vi "Main.vi"() -> ()   [LabVIEW 2018]
uses:
  <vilib>/addons/database/Connection.llb/DB Tools Open Connec (String).vi
  <vilib>/addons/database/NI_Database_API.lvlib
  <vilib>/ptbypt/NI_PtbyPt.lvlib
panel:
  out "元素":cluster{"Data":string[], "State":T1}
  out "Code":string
  out "退出":bool
  out "Main Tab":T2(tab)
  out "ST80通讯状态":bool caption="ST60通讯状态"
  in  "错误信息":i32(listbox)
  out "ST30通讯状态":bool caption="ST10通讯状态"
  out "ST50通讯状态":bool
  out "ST70通讯状态":bool caption="ST60通讯状态"
  out "ST60通讯状态":bool caption="ST70通讯状态"
  out "ST40通讯状态":bool
  out "ST20通讯状态":bool
  out "ST10通讯状态":bool
  in  "每工站主要显示":T3(tab)
  in  "ST10-2_DATA":i32(listbox) caption="ST10_DATA"
  in  "ST10-1_DATA":i32(listbox) caption="ST10_DATA"
  in  "ST20-3_DATA":i32(listbox) caption="ST20_DATA"
  in  "ST20-2_DATA":i32(listbox) caption="ST20_DATA"
  in  "ST30-2_DATA":i32(listbox) caption="ST20_DATA"
  in  "ST30-1_DATA":i32(listbox) caption="ST20_DATA"
  in  "ST40-3_DATA":i32(listbox) caption="ST20_DATA"
  in  "ST40-1_DATA":i32(listbox) caption="ST20_DATA"
  in  "ST50-3_DATA":i32(listbox) caption="ST20_DATA"
  in  "ST50-2_DATA":i32(listbox) caption="ST20_DATA"
  in  "ST60-2_DATA":i32(listbox) caption="ST20_DATA"
  in  "ST60-1_DATA":i32(listbox) caption="ST20_DATA"
  in  "ST70_DATA":i32(listbox) caption="ST20_DATA"
  out "XY图":cluster{"X":dbl, "Y":dbl}[](graph)
  in  "登录界面":bool
  in  "注销":bool
  in  "修改密码":bool
  in  "Rework界面":bool
  out "产品型号":string
  in  "界面切换":bool
  in  "登录界面返回":bool
  out "登录状态":string
  in  "登录":bool
  in  "输入管理员密码":string
  in  "修改密码界面返回":bool
  out "修改密码状态":string
  in  "确认修改密码":bool
  in  "新密码":string
  in  "初始密码":string
  in  "80":bool
  in  "602":bool
  in  "403":bool
  in  "302":bool
  in  "203":bool
  in  "101":bool
  out "Rework状态":string
  in  "查询":bool
  in  "确定Rework":bool
  in  "Rework返回":bool
  in  "输入需要Rework的一维码：":string
  in  "102":bool
  in  "202":bool
  in  "301":bool
  in  "401":bool
  in  "502":bool
  in  "503":bool
  in  "601":bool
  in  "70":bool
  in  "Monitor Tab":T4(tab)
  out "202读取数据":string[](array[string])
  out "ST102数据读取（事件）":bool
  out "ST10 Shaft M0102049":string caption="ST101 Shaft M0102049"
  out "数据保存请求回复101":string
  out "扫码请求回复102":string
  out "上一站结果(102)":string
  out "上一站号(102)":string
  out "ST102扫码请求":bool
  out "ST101扫码请求":bool
  out "ST101数据读取":bool
  out "扫码请求回复101":string
  in  "ST102扫码请求（事件）":bool
  out "ST101扫码请求（事件）":bool
  out "ST101数据读取（事件）":bool
  in  "返回":bool
  out "ST102数据读取":bool
  out "数据保存请求回复102":string
  out "101 二维码":string
  out "102 二维码":string
  out "ST10 Form Seal 5026859":string caption="ST101 Form Seal 5026859"
  out "ST10 Dowel Pin 5024532":string caption="ST101 Dowel Pin 5024532"
  out "ST10 Flange M0104918":string caption="ST101 Flange M0104918"
  out "ST10 Control Plat 5025303":string caption="ST101 Control Plat 5025303"
  out "ST10 Dowel Pin 5020281":string caption="ST101 Dowel Pin 5020281"
  out "ST203扫码请求":bool
  out "202二维码":string caption="203二维码"
  out "ST203扫码请求（事件）":bool
  out "扫码请求回复202":string caption="扫码请求回复203"
  out "ST202数据读取":bool caption="ST203数据读取"
  out "ST203数据读取（事件）":bool
  out "数据保存请求回复202":string caption="数据保存请求回复203"
  out "ST202 Dowel Pin M0104893":string caption="ST20 Dowel Pin M0104893"
  out "ST202 Camring 5026187":string caption="ST20 Camring 5026187"
  out "ST202 Rotor 5025805":string caption="ST20 Rotor 5025805"
  out "201二维码":string caption="202二维码"
  out "上一站号 (202)":string
  out "上一站结果 (202)":string
  out "扫码请求回复201":string caption="扫码请求回复202"
  out "数据保存请求回复201":string caption="数据保存请求回复202"
  out "ST201数据读取":bool caption="ST202数据读取"
  out "ST202扫码请求":bool
  out "ST202扫码请求(事件)":bool
  in  "ST202数据读取(事件)":bool
  out "上一站结果 (203)":string
  out "上一站号 (203)":string
  out "State 10":T1
  out "10":i32
  out "20":i32
  out "20 State":T1
  out "101 上一站号":string
  out "101 上一站结果":string
  out "102读取数据":string[](array[string])
  out "数据库连接状态":string="连接成功"
  out "403读取数据":string[](array[string])
  out "302读取数据":string[](array[string])
  out "301 二维码":string
  out "302 二维码":string
  out "ST301扫码请求":bool
  out "上一站号 (301)":string
  out "上一站结果 (301)":string
  out "ST301数据读取 (事件)":bool
  out "ST301扫码请求 (事件)":bool
  out "ST302数据读取 (事件)":bool
  out "ST302扫码请求 (事件)":bool
  out "扫码请求回复301":string
  out "ST301数据读取":bool
  out "数据保存请求回复301":string
  out "ST302扫码请求":bool
  out "扫码请求回复302":string
  out "ST302数据读取":bool
  out "ST301 Vane 5004737":string caption="ST30 Vane 5004737"
  out "ST301 Dowel Pin 5024533":string caption="ST30 Dowel Pin 5024533"
  out "ST301 Dowel Pin 5020282":string caption="ST30 Dowel Pin 5020282"
  out "数据保存请求回复302":string
  out "401二维码":string
  out "402二维码 2":string caption="402二维码"
  out "403二维码":string
  out "ST401扫码请求":bool
  out "扫码请求回复401":string
  out "ST401数据读取":bool
  out "数据保存请求回复401":string
  out "ST402扫码请求":bool
  out "扫码请求回复402":string
  out "ST402数据读取":bool
  out "数据保存请求回复402":string
  out "ST403扫码请求":bool
  out "扫码请求回复403":string
  out "ST403数据读取":bool
  out "数据保存请求回复403":string
  out "ST403数据读取（事件）":bool
  out "ST403扫码请求(事件)":bool
  out "ST401数据读取（事件）":bool
  out "ST401扫码请求(事件)":bool
  out "ST402数据读取（事件）":bool
  out "ST402扫码请求(事件)":bool caption="ST402扫码请求（事件）"
  out "上一站号 (401)":string
  out "上一站结果 (401)":string
  out "ST40 Circlip 5026621":string
  out "上一站结果 (302)":string
  out "上一站号 (302)":string
  out "上一站结果 (403)":string
  out "上一站号 (403)":string
  out "30_State":T1
  out "30":i32
  out "40_State":T1
  out "40":i32
  out "602读取数据":string[](array[string])
  out "503读取数据":string[](array[string])
  out "ST502 Pressure Plate M0105053":string caption="ST50 Pressure Plate M0105053"
  out "ST502 O-Ring M0104976":string caption="ST50 O-Ring M0104976"
  out "ST502 Support Ring 5027083":string caption="ST50 Support Ring 5027083"
  out "ST502 Form Seal 5026860":string caption="ST50 Form Seal 5026860"
  out "502二维码":string
  out "503二维码":string
  out "上一站号 (503)":string
  out "上一站结果 (503)":string
  out "数据保存请求回复502":string caption="数据保存请求回复503"
  out "扫码请求回复502":string caption="扫码请求回复503"
  out "ST503数据读取（事件）":bool
  out "ST502数据读取":bool caption="ST503数据读取"
  out "ST503扫码请求(事件)":bool
  out "ST502扫码请求":bool caption="ST503扫码请求"
  out "上一站号 (502)":string
  out "上一站结果 (502)":string
  out "数据保存请求回复501":string caption="数据保存请求回复502"
  out "扫码请求回复501":string caption="扫码请求回复502"
  out "ST502数据读取（事件）":bool
  out "ST502扫码请求(事件)":bool
  out "ST501数据读取":bool caption="ST502数据读取"
  out "ST501扫码请求":bool caption="ST502扫码请求"
  out "ST60 Eclip 5018568":string
  out "ST60 Sleeve 5020302":string
  out "ST60 Disk Spring 5024300":string
  out "ST601扫码请求":bool
  out "601二维码":string
  out "ST601数据读取":bool
  out "扫码请求回复601":string
  out "数据保存请求回复601":string
  out "ST602扫码请求":bool
  out "ST602数据读取":bool
  out "ST602扫码请求(事件)":bool
  out "ST602数据读取(事件)":bool
  out "扫码请求回复602":string
  out "数据保存请求回复602":string
  out "602二维码":string
  out "ST601数据读取（事件）":bool
  out "ST601扫码请求(事件)":bool
  out "上一站结果 (601)":string
  out "上一站号 (601)":string
  out "上一站结果 (602)":string
  out "上一站号 (602)":string
  out "50":i32
  out "50_State":T1
  out "60":i32
  out "60_State":T1
  out "802查询条件":string caption="查询条件"
  out "80保存回复":string
  out "ST802保存数据(事件)":bool
  out "上一站结果 (802)":string
  out "上一站号 (802)":string
  out "ST802扫码请求":bool
  out "ST802扫码请求(事件)":bool
  out "80产品型号":u32
  out "刻印码 16":string
  out "OP70画曲线":bool
  out "ST70 Shaft Seal 5024366":string
  out "上一站号 (70)":string
  out "上一站结果 (70)":string
  out "数据保存请求回复70":string
  out "扫码请求回复70":string
  out "70二维码":string
  out "ST70数据读取":bool
  out "ST70扫码请求":bool
  out "ST70数据读取(事件)":bool
  out "ST70扫码请求(事件)":bool
  out "70":i32
  out "70_State":T1
  out "刻印码":string
  out "曲线文件路径":path
  out "error IO":errorcluster
  out "80_State":T1
  out "ST80扫码请求":bool
  out "80二维码":string
  out "扫码请求回复80":string
  out "80":i32
  out "ST80扫码请求(事件)":bool
  out "上一站结果 (80)":string
  out "上一站号 (80)":string
  out "数据":u32[](array[numeric])
  out "802二维码":string
  out "ST802保存数据":bool caption="ST802保存数据请求"
  out "802数据":string[](array[string])
  # "数据库追溯系统"
  # "报警提示"
  # "V1.0"
  # "登 录"
  # "修 改 密 码"
  # "Rework"
  # "ST20"
  # "ST10"
  # "ST30"
  # "ST40"
  # "ST60"
  # "ST50"
  # "ST70"
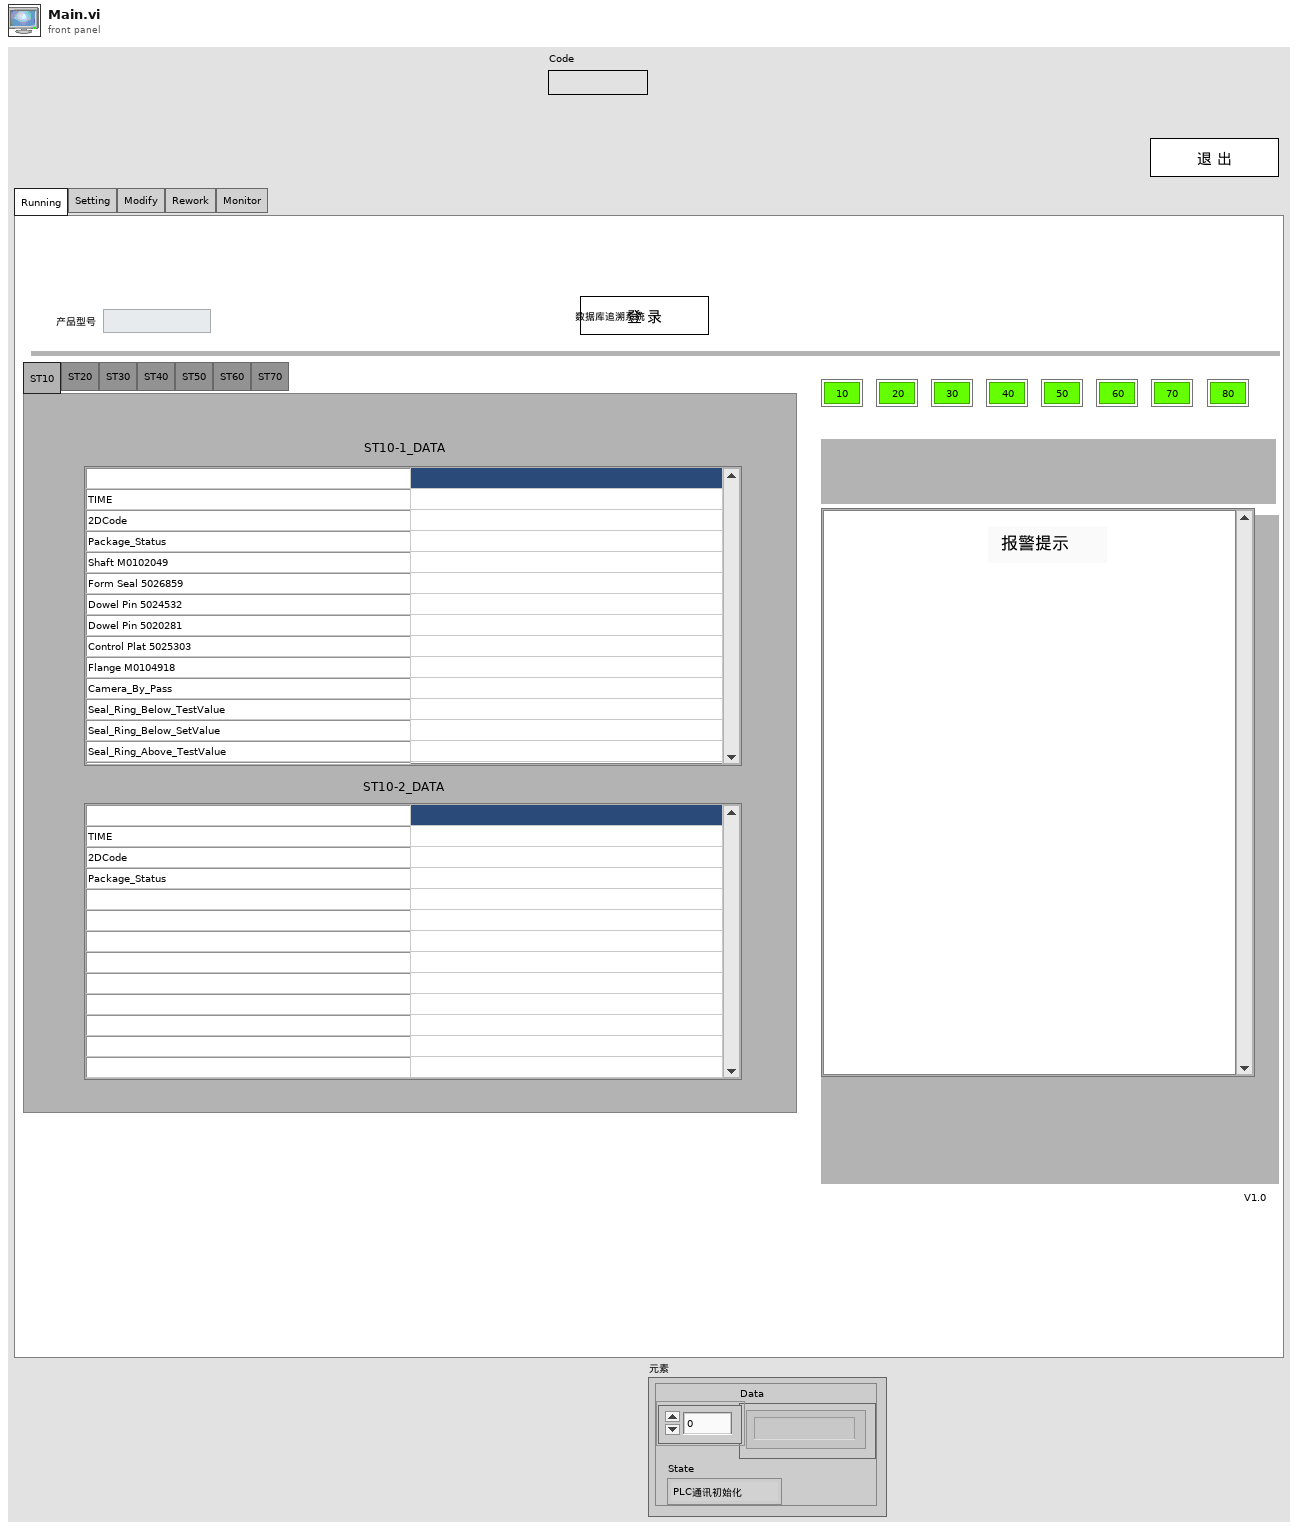
[diagram p1: front panel]
types:
  T1 = typedef "状态2.ctl" = enum16{"PLC通讯初始化", "---------------", "读左扫码请求", "读左二维码", "10左扫码回复", "--------------", "读扫码请求", "读二维码", "扫码回复", "-------------", "读数据保存请求", "读数据", "数据保存回复", "-----------------", "错误", "退出", "-------------------", "读扫码请求2", "读二维码2", "扫码回复2", "-- --------------", "读数据保存请求2", "读数据2", "数据保存回复2", "------------", "读扫码请求3", "读二维码3", "扫码回复3", "- ---------", "读数据保存请求3", "读数据3", "数据保存回复3", "----------", "看门狗", "------  --", "读料号请求1", "读料号1", "回复料号请求1", "--- ---- -", "读料号请求2", "读料号2", "回复料号请求2", "---- --------", "读料号请求3", "读料号3", "回复料号请求3", "-- - -  ------", "读料号请求4", "读料号4", "回复料号请求4", "---------- ---", "读PartNumber请求1", "读PartNumber1", "回复PartNumber请求1", "---------- ------", "读PartNumber请求2", "读PartNumber2", "回复PartNumber请求2", "---- -------------", "读PartNumber请求3", "读PartNumber3", "回复PartNumber请求3", "----------- ------", "读PartNumber请求4", "读PartNumber4", "回复PartNumber请求4"}
  T2 = enum32{"Running", "Setting", "Modify", "Rework", "Monitor"}
  T3 = enum32{"ST10", "ST20", "ST30", "ST40", "ST50", "ST60", "ST70"}
  T4 = enum32{"Interface 1", "Interface 2", "Interface 3", "Interface 4"}
  T5 = cluster{"扫码超时":string, "数据保存超时":string, "看门狗":string, "扫码超时 2":string}
  T6 = enum32{"Invalid", "Standard", "Closed", "Hidden", "Minimized", "Maximized"}
  T7 = cluster{"扫码超时1":string, "数据保存超时1":string, "扫码超时2":string, "数据保存超时2":string, "看门狗":string, "扫码超时3":string, "数据保存超时3":string, "条码":string, "次数":i32}
  T8 = cluster{"扫码2超时":string, "扫码1超时":string, "数据保存1超时":string, "看门狗":string, "数据保存2超时":string}
  T9 = cluster{"扫码超时1":string, "数据保存超时1":string, "扫码超时2":string, "数据保存超时2":string, "看门狗":string}
  T10 = cluster{"扫码超时":string, "数据保存超时":string, "看门狗":string}
  T11 = cluster{"扫码超时1":string, "数据保存超时1":string, "看门狗":string, "扫码超时2":string, "数据保存超时2":string}
  T12 = typedef "NI_Database_API.lvlib/Conn ObjectReference.ctl" = refnum<k1>
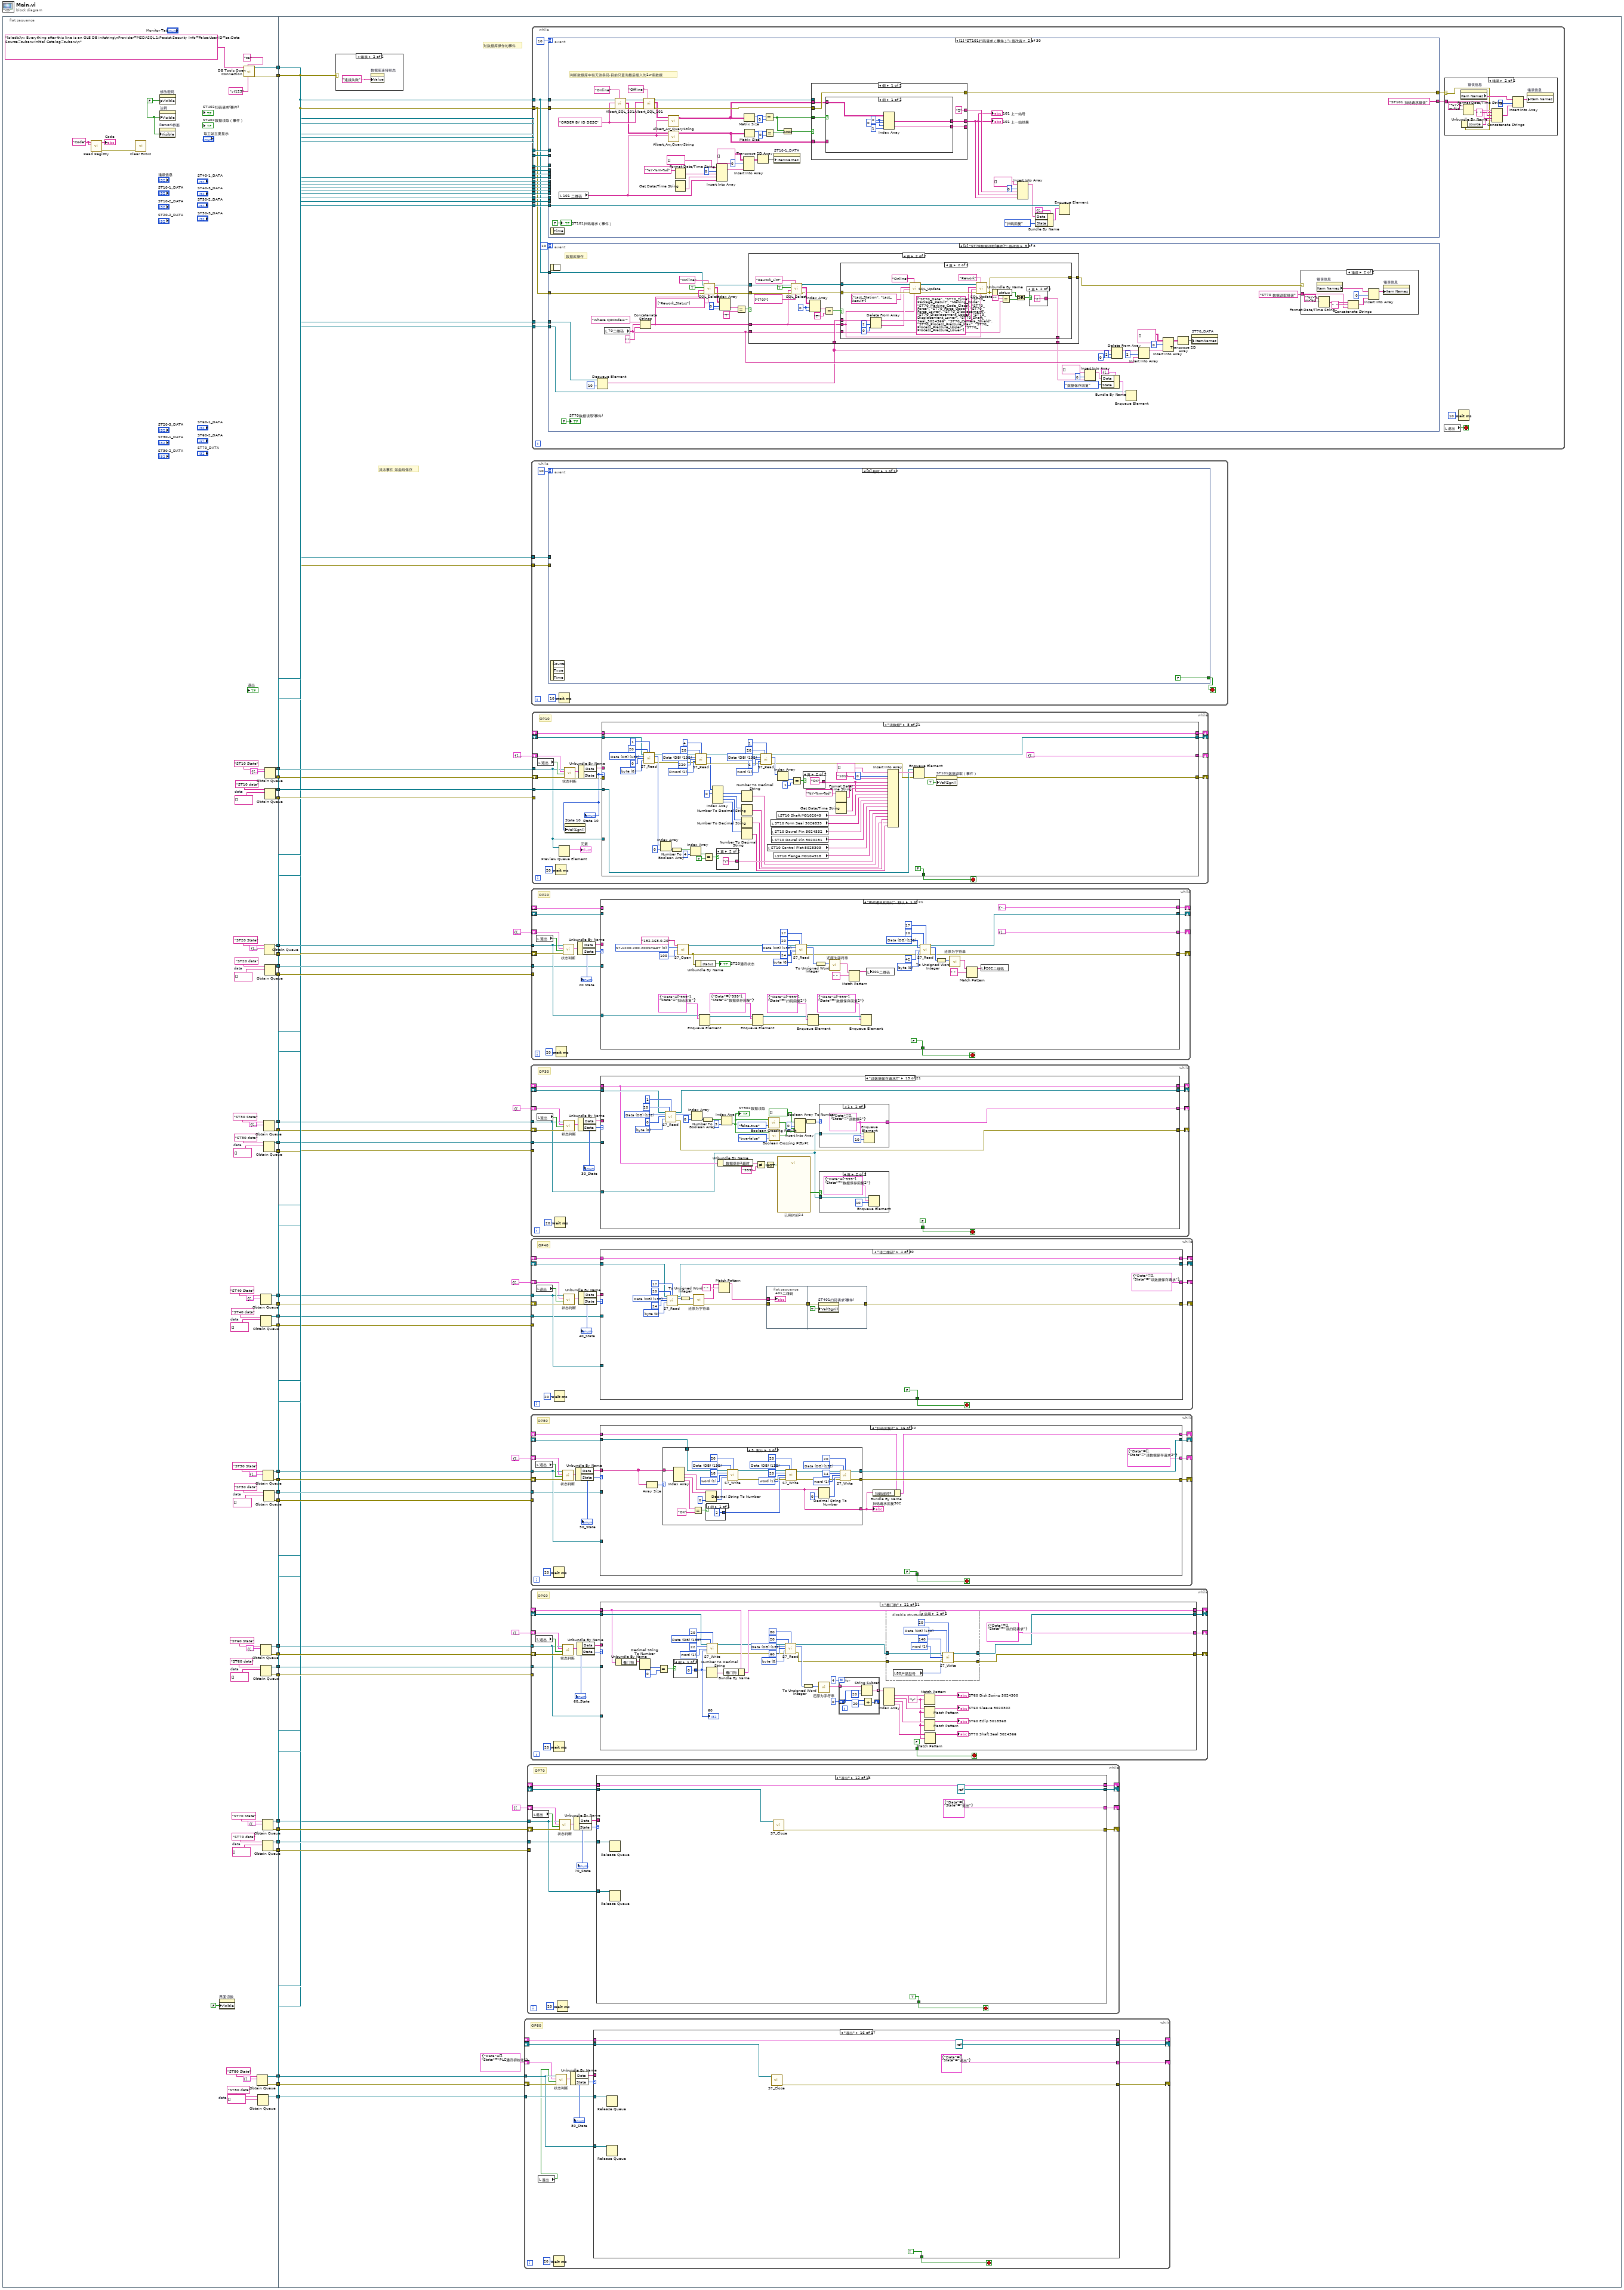
[diagram p0: block diagram]
diagram:
  n1 = flat-sequence {
    tunnel: [w42] -> w33
    tunnel: [w41] -> w32
    tunnel: [w102] -> w31
    tunnel: [w101] -> w30
    tunnel: [w100] -> w29
    tunnel: [w99] -> w28
    tunnel: [w93] -> w27
    tunnel: [w94] -> w26
    tunnel: [w92] -> w25
    tunnel: [w91] -> w24
    tunnel: [w86] -> w23
    tunnel: [w85] -> w22
    tunnel: [w84] -> w21
    tunnel: [w83] -> w20
    tunnel: [w78] -> w19
    tunnel: [w77] -> w18
    tunnel: [w76] -> w17
    tunnel: [w75] -> w16
    tunnel: [w70] -> w15
    tunnel: [w69] -> w14
    tunnel: [w68] -> w13
    tunnel: [w67] -> w12
    tunnel: [w62] -> w11
    tunnel: [w61] -> w10
    tunnel: [w60] -> w9
    tunnel: [w59] -> w8
    tunnel: [w54] -> w7
    tunnel: [w53] -> w6
    tunnel: [w52] -> w5
    tunnel: [w51] -> w4
    tunnel: [w45] -> w3
    tunnel: [w44] -> w2
    tunnel: [w43] -> w1
    tunnel: w33 -> [w144]
    tunnel: w32 -> [w107]
    tunnel: w31 -> [w108]
    tunnel: w30 -> [w147]
    tunnel: w29 -> [w146]
    tunnel: w28 -> [w145]
    tunnel: w27 -> [w141]
    tunnel: w26 -> [w143]
    tunnel: w25 -> [w140]
    tunnel: w24 -> [w142]
    tunnel: w23 -> [w124]
    tunnel: w22 -> [w125]
    tunnel: w21 -> [w123]
    tunnel: w20 -> [w122]
    tunnel: w19 -> [w120]
    tunnel: w18 -> [w119]
    tunnel: w17 -> [w118]
    tunnel: w16 -> [w117]
    tunnel: w15 -> [w137]
    tunnel: w14 -> [w139]
    tunnel: w13 -> [w136]
    tunnel: w12 -> [w138]
    tunnel: w11 -> [w109]
    tunnel: w10 -> [w135]
    tunnel: w9 -> [w116]
    tunnel: w8 -> [w134]
    tunnel: w7 -> [w115]
    tunnel: w6 -> [w133]
    tunnel: w5 -> [w114]
    tunnel: w4 -> [w132]
    tunnel: w3 -> [w111]
    tunnel: w2 -> [w112]
    tunnel: w1 -> [w110]
    frame #0 {
      w34 = "Code" ("subkeyName")
      w46 = string[] []  # data
      w50 = FALSE ("可见")
      w55 = string[] []  # data
      w66 = string[] []  # data
      w74 = string[] []  # data
      w82 = string[] []  # data
      w90 = string[] []  # data
      w95 = string[] []  # data
      w106 = string[] []  # data
      n2 = call "Read Registry.vi"("value"=w34, "subkeyName"=w34) -> ("error out"=w36:errorcluster, "Data"=→"Code":string)  [unwired: 6 in]
      n3 = call <vilib>:"Clear Errors.vi"("error in (no error)"=w36) -> ()  [unwired: 5 in, 2 out]
      n4 = property on="Rework界面" class="Bool"("Visible"=w50) -> ()  [unwired: 2 in, 2 out]
      n5 = property on="修改密码" class="Bool"("Visible"=w50) -> ()  [unwired: 2 in, 2 out]
      n6 = property on="注销" class="Bool"("Visible"=w50) -> ()  [unwired: 2 in, 2 out]
      n7 = property on="界面切换" class="Bool (严格)"("Visible"=FALSE ("可见")) -> ()  [unwired: 2 in, 2 out]
      n8 = call-poly <vilib>:"DB Tools Open Connection.vi"("password"="yt123", "userID"="sa", "connection information"="[oledb]\n; Everything after this line is an OLE DB initstring\nProvider=MSDASQL.1;Persist Security Info=False;User ID=sa;Data Source=subaru;Initial Catalog=subaru\n") -> ("error out"=w41:errorcluster, "connection reference"=w42:T12)  [unwired: 5 in]
      n9 = Obtain Queue(name (unnamed)="ST80 State" ("名称（未命名）"), element data type=cluster{"Data":string[], "State":T1} {"Data"=[], "State"=enum."PLC通讯初始化"} ("簇")) -> (queue out=w45:refnum<queue>, error out=w44:errorcluster)  [unwired: 3 in, 1 out]
      n10 = Obtain Queue(name (unnamed)="ST80 data" ("名称（未命名）"), element data type=w46) -> (queue out=w43:refnum<queue>)  [unwired: 3 in, 2 out]
      n11 = Obtain Queue(name (unnamed)="ST40 State" ("名称（未命名）"), element data type=cluster{"Data":string[], "State":T1} {"Data"=[], "State"=enum."PLC通讯初始化"} ("簇")) -> (queue out=w78:refnum<queue>, error out=w77:errorcluster)  [unwired: 3 in, 1 out]
      n12 = Obtain Queue(name (unnamed)="ST60 State" ("名称（未命名）"), element data type=cluster{"Data":string[], "State":T1} {"Data"=[], "State"=enum."PLC通讯初始化"} ("簇")) -> (queue out=w54:refnum<queue>, error out=w53:errorcluster)  [unwired: 3 in, 1 out]
      n13 = Obtain Queue(name (unnamed)="ST40 data" ("名称（未命名）"), element data type=w82) -> (queue out=w76:refnum<queue>, error out=w75:errorcluster)  [unwired: 3 in, 1 out]
      n14 = Obtain Queue(name (unnamed)="ST60 data" ("名称（未命名）"), element data type=w55) -> (queue out=w52:refnum<queue>, error out=w51:errorcluster)  [unwired: 3 in, 1 out]
      n15 = Obtain Queue(name (unnamed)="ST70 State" ("名称（未命名）"), element data type=cluster{"Data":string[], "State":T1} {"Data"=[], "State"=enum."PLC通讯初始化"} ("簇")) -> (queue out=w62:refnum<queue>, error out=w61:errorcluster)  [unwired: 3 in, 1 out]
      n16 = Obtain Queue(name (unnamed)="ST70 data" ("名称（未命名）"), element data type=w66) -> (queue out=w60:refnum<queue>, error out=w59:errorcluster)  [unwired: 3 in, 1 out]
      n17 = Obtain Queue(name (unnamed)="ST50 State" ("名称（未命名）"), element data type=cluster{"Data":string[], "State":T1} {"Data"=[], "State"=enum."PLC通讯初始化"} ("簇")) -> (queue out=w70:refnum<queue>, error out=w69:errorcluster)  [unwired: 3 in, 1 out]
      n18 = Obtain Queue(name (unnamed)="ST30 State" ("名称（未命名）"), element data type=cluster{"Data":string[], "State":T1} {"Data"=[], "State"=enum."PLC通讯初始化"} ("簇")) -> (queue out=w85:refnum<queue>, error out=w86:errorcluster)  [unwired: 3 in, 1 out]
      n19 = Obtain Queue(name (unnamed)="ST50 data" ("名称（未命名）"), element data type=w74) -> (queue out=w68:refnum<queue>, error out=w67:errorcluster)  [unwired: 3 in, 1 out]
      n20 = Obtain Queue(name (unnamed)="ST30 data" ("名称（未命名）"), element data type=w90) -> (queue out=w84:refnum<queue>, error out=w83:errorcluster)  [unwired: 3 in, 1 out]
      n21 = Obtain Queue(name (unnamed)="ST20 State" ("名称（未命名）"), element data type=cluster{"Data":string[], "State":T1} {"Data"=[], "State"=enum."PLC通讯初始化"} ("簇")) -> (queue out=w93:refnum<queue>, error out=w94:errorcluster)  [unwired: 3 in, 1 out]
      n22 = Obtain Queue(name (unnamed)="ST10 State" ("名称（未命名）"), element data type=cluster{"Data":string[], "State":T1} {"Data"=[], "State"=enum."PLC通讯初始化"} ("簇")) -> (queue out=w101:refnum<queue>, error out=w102:errorcluster)  [unwired: 3 in, 1 out]
      n23 = Obtain Queue(name (unnamed)="ST20 data" ("名称（未命名）"), element data type=w95) -> (queue out=w92:refnum<queue>, error out=w91:errorcluster)  [unwired: 3 in, 1 out]
      n24 = Obtain Queue(name (unnamed)="ST10 data" ("名称（未命名）"), element data type=w106) -> (queue out=w99:refnum<queue>, error out=w100:errorcluster)  [unwired: 3 in, 1 out]
    }
    frame #1 {
      # "对数据库操作的事件"
      # "其余事件 如曲线保存"
      n25 = case shown="错误" w107 {
        frame No Error {
          "数据库连接状态" <- "连接成功"
        }
        frame Error {
          n26 = property on="数据库连接状态" class="Str"("Value"="连接失败") -> ()  [unwired: 2 in, 2 out]
        }
      }
      n27 = while {
        shift-right: [w156] -> _
        shift-left: cluster{"Data":string[], "State":T1} {"Data"=[], "State"=enum."PLC通讯初始化"} ("元素") -> [w157]
        shift-right: [w164] -> _
        shift-left: w112 -> [w161]
        shift-right: [w165] -> _
        shift-left: _ -> [w162]
        tunnel: w111 -> [w158]
        tunnel: w110 -> [w153]
        shift-right: [w152] -> _
        shift-left: _ -> [w151]
        stop <- w154 stop-if-true
        # "OP80"
        n28 = local read "退出"() -> (w150:bool)
        n29 = Wait (ms)(milliseconds to wait=u32 20 ("等待时间（毫秒）")) -> ()  [unwired: 1 out]
        n30 = call "状态判断.vi"("error IO"=w161, "退出？"=w150, "簇 输入"=w157, "队列输入"=w158) -> ("簇"=w160:cluster{"Data":string[], "State":T1})  [unwired: 6 in, 1 out]
        n31 = Unbundle By Name(w160) -> ("Data"=w155:string[], "State"=w159:T1)
        "80_State" <- w159
        n32 = case shown="\"退出\"" w159 {
          tunnel: [w167 w181 w203 w238 w260 w311 w331 w366 w388 w438 w459 w495 w534 w551 refnum<k5> refnum ("TCP") refnum<k5> refnum ("TCP") w572] -> w165
          tunnel: [w166 errorcluster {"status"=FALSE, "code"=0, "source"=""} ("error out") w182 w234 w254 errorcluster {"status"=FALSE, "code"=0, "source"=""} ("error out") w315 w359 w383 errorcluster {"status"=FALSE, "code"=0, "source"=""} ("error out") w443 w482 w533 errorcluster {"status"=FALSE, "code"=0, "source"=""} ("error out") errorcluster {"status"=FALSE, "code"=0, "source"=""} ("error out") w562 w570] -> w164
          tunnel: w162 -> [_ w181 w204 w233 w261 w311 w332 w362 w389 w438 w460 w509 w537 w551 w559 w565 w580]
          tunnel: w158 -> [w170 _ w186 _ _ _ w317 _ _ _ w445 _ _ _ w555 w566 _]
          tunnel: [cluster{"Data":string[], "State":T1} {"Data"=[], "State"=enum."读扫码请求"} ("元素") cluster{"Data":string[], "State":T1} {"Data"=[], "State"=enum."读扫码请求"} ("元素") w193 cluster{"Data":string[], "State":T1} {"Data"=[], "State"=enum."读扫码请求2"} ("元素") cluster{"Data":string[], "State":T1} {"Data"=[], "State"=enum."读扫码请求2"} ("元素") cluster{"Data":string[], "State":T1} {"Data"=[], "State"=enum."读扫码请求2"} ("元素") w323 cluster{"Data":string[], "State":T1} {"Data"=[], "State"=enum."读数据保存请求2"} ("元素") cluster{"Data":string[], "State":T1} {"Data"=[], "State"=enum."读数据保存请求2"} ("元素") cluster{"Data":string[], "State":T1} {"Data"=[], "State"=enum."读数据保存请求2"} ("元素") w451 cluster{"Data":string[], "State":T1} {"Data"=[], "State"=enum."数据保存回复2"} ("元素") cluster{"Data":string[], "State":T1} {"Data"=[], "State"=enum."看门狗"} ("元素") cluster{"Data":string[], "State":T1} {"Data"=[], "State"=enum."看门狗"} ("元素") cluster{"Data":string[], "State":T1} {"Data"=[], "State"=enum."PLC通讯初始化"} ("元素") cluster{"Data":string[], "State":T1} {"Data"=[], "State"=enum."退出"} ("元素") cluster{"Data":string[], "State":T1} {"Data"=[], "State"=enum."读扫码请求"} ("元素")] -> w156
          tunnel: w155 -> [_ _ _ _ w258 _ _ _ w386 _ _ _ w536 _ _ _ _]
          tunnel: [FALSE FALSE FALSE FALSE FALSE FALSE FALSE FALSE FALSE FALSE FALSE FALSE FALSE FALSE FALSE TRUE FALSE] -> w154
          tunnel: w153 -> [_ _ _ _ _ _ _ _ _ _ _ _ _ _ w556 w567 _]
          tunnel: [T5 {"扫码超时"="999", "数据保存超时"="999", "看门狗"="999", "扫码超时 2"="999"} w178 w185 w235 w256 w308 w316 w363 w384 w439 w444 w510 w544 w552 w554 w563 w574] -> w152
          tunnel: w151 -> [_ w178 w185 w235 w257 w308 w316 w363 w385 w439 w444 w510 w545 w552 w554 w563 w575]
          frame "PLC通讯初始化", Default {
            w175 = u8 0 items=["S7-1200.200.200SMART"=0, "S7-300"=2, "S7-400"=3] ("PLC 系列")
            n33 = Enqueue Element(queue=w170, element=cluster{"Data":string[], "State":T1} {"Data"=["999"], "State"=enum."扫码回复"} ("元素")) -> ()  [unwired: 2 in, 3 out]
            n34 = call "S7_Open.vi"("IP 地址"="192.168.0.80", "PLC 系列"=w175, "超时（MS）"=100) -> ("TCP"=w167:refnum<k5>, "error out"=w166:errorcluster)  [unwired: 10 in, 1 out]
            n35 = Unbundle By Name(w166) -> ("status"=→"ST80通讯状态":bool)
          }
          frame "--------------" {
          }
          frame "读扫码请求" {
            w212 = u16 0 items=["byte", "word", "Dword"] ("数据类型")
            w214 = u8 132 items=["I/O (P)"=128, "Input (I)"=129, "Output (Q)"=130, "Bit Memory (M)"=131, "Data (DB)"=132, "Instance Data (DI)"=133, "Local Data (L)"=134, "Predecessor Local Data (VL)"=135] ("寄存器类型")
            n36 = call "S7_Read.vi"("TCP"=w204, "DB #"=u16 20, "读取长度"=u16 1, "寄存器类型"=w214, "起始地址"=u32 0, "数据类型"=w212) -> ("TCP"=w203:refnum<k5>, "数据"=w209:u32[], "读取成功"=w183:bool, "error out"=w182:errorcluster)  [unwired: 6 in]
            n37 = Not(x=w183) -> (.not. x?=w184:bool)
            n38 = local write "ST80通讯状态"(w184) -> ()
            n39 = Index Array(array=w209, index=0 ("索引")) -> (element=w207:u32)
            n40 = Number To Boolean Array(number=w207) -> (Boolean array=w206:bool[])
            n41 = Index Array(array=w206, index=0 ("索引")) -> (element=w192:bool)
            "ST80扫码请求" <- w192
            n42 = Unbundle By Name(w185) -> ("扫码超时"=w187:string)
            n43 = Not Equal?(x=w187, y="999") -> (x != y?=w189:bool)
            n44 = call <vilib>:"Boolean Crossing PtByPt.vi"("direction"=enum16{"either", "false-true", "true-false"}."false-true", "input"=w192) -> ("crossing"=w199:bool)  [unwired: 1 in]
            n45 = call <vilib>:"Boolean Crossing PtByPt.vi"("direction"=enum16{"either", "false-true", "true-false"}."true-false", "input"=w192) -> ("crossing"=w198:bool)  [unwired: 1 in]
            n46 = Not(x=w189) -> (.not. x?=w190:bool)
            n47 = call "已用时间29"("Reset"=w190) -> ("Time has Elapsed"=w191:bool)  [unwired: 11 in, 7 out]
            n48 = Insert Into Array(array=bool[] [] ("数组"), index=0 ("索引"), new element #1=w199, new element #2=w198) -> (w195:bool[])
            n49 = Boolean Array To Number(Boolean array=w195) -> (number=w194:u32)
            n50 = case shown="0, 默认" w194 {
              tunnel: [cluster{"Data":string[], "State":T1} {"Data"=[], "State"=enum."读扫码请求2"} ("元素") w219 w223] -> w193
              tunnel: w186 -> [_ w220 w224]
              frame 0, Default {
              }
              frame 1 {
                w219 = cluster{"Data":string[], "State":T1} {"Data"=[], "State"=enum."读二维码"} ("元素")
                n51 = Enqueue Element(queue=w220, element=w219, timeout in ms (-1)=10 ("超时毫秒(-1)")) -> ()  [unwired: 1 in, 3 out]
              }
              frame 2 {
                w223 = cluster{"Data":string[], "State":T1} {"Data"=["999"], "State"=enum."扫码回复"} ("元素")
                n52 = Enqueue Element(queue=w224, element=w223, timeout in ms (-1)=10 ("超时毫秒(-1)")) -> ()  [unwired: 1 in, 3 out]
              }
            }
            n53 = case shown="真" w191 {
              tunnel: w186 -> [_ w216]
              frame False {
              }
              frame True {
                n54 = Enqueue Element(queue=w216, element=cluster{"Data":string[], "State":T1} {"Data"=["999"], "State"=enum."扫码回复"} ("元素"), timeout in ms (-1)=10 ("超时毫秒(-1)")) -> ()  [unwired: 1 in, 3 out]
              }
            }
          }
          frame "读二维码" {
            w243 = u16 0 items=["byte", "word", "Dword"] ("数据类型")
            w239 = u8 132 items=["I/O (P)"=128, "Input (I)"=129, "Output (Q)"=130, "Bit Memory (M)"=131, "Data (DB)"=132, "Instance Data (DI)"=133, "Local Data (L)"=134, "Predecessor Local Data (VL)"=135] ("寄存器类型")
            n55 = call "S7_Read.vi"("TCP"=w233, "DB #"=u16 20, "读取长度"=u16 17, "寄存器类型"=w239, "起始地址"=u32 10, "数据类型"=w243) -> ("TCP"=w238:refnum<k5>, "数据"=w244:u32[], "读取成功"=w231:bool, "error out"=w246:errorcluster)  [unwired: 6 in]
            n56 = Not(x=w231) -> (.not. x?=w232:bool)
            n57 = To Unsigned Word Integer(number=w244) -> (unsigned 16bit integer=w245:u16[])
            n58 = local write "ST80通讯状态"(w232) -> ()
            n59 = call "还原为字符串.vi"("error in (no error)"=w246, "输入数组"=w245) -> ("error out"=w230:errorcluster, "字符串"=w226:string)  [unwired: 8 in]
            n60 = disable-structure shown="禁用" {
              frame Disabled {
                n61 = String Subset(offset (0)=0 ("偏移量(0)"), length (rest)=13 ("长度（剩余）")) -> ()  [unwired: 1 in, 1 out]
              }
              frame Enabled {
              }
            }
            n62 = String Subset(string=w226, offset (0)=0 ("偏移量(0)"), length (rest)=13 ("长度（剩余）")) -> (substring=w225:string)
            n63 = flat-sequence {
              tunnel: w230 -> [w250]
              tunnel: [w250] -> w229
              tunnel: w225 -> [w249]
              tunnel: [w252] -> w234
              tunnel: w229 -> [w251]
              frame #0 {
                "80二维码" <- w249
              }
              frame #1 {
                n64 = property on="ST80扫码请求(事件)" class="Bool (严格)"(error in=w251, "Val(Sgnl)"=TRUE ("值(信号)")) -> (error out=w252:errorcluster)  [unwired: 1 in, 1 out]
              }
            }
          }
          frame "扫码回复" {
            n65 = Array Size(array=w258) -> (size(s)=w259:i32)
            n66 = case shown="1" w259 {
              tunnel: w258 -> [w266 w299]
              tunnel: w261 -> [w265 w286]
              tunnel: [w267 w277] -> w260
              tunnel: [w268 w276] -> w254
              tunnel: [w264 w275] -> w255
              frame 1 {
                w271 = u8 132 items=["I/O (P)"=128, "Input (I)"=129, "Output (Q)"=130, "Bit Memory (M)"=131, "Data (DB)"=132, "Instance Data (DI)"=133, "Local Data (L)"=134, "Predecessor Local Data (VL)"=135] ("寄存器类型")
                w270 = u16 1 items=["byte", "word", "Dword"] ("数据类型")
                n67 = Index Array(array=w266) -> (element=w264:string)  [unwired: 1 in]
                n68 = Decimal String To Number(string=w264, default (0L)=u32 0 ("默认(0 I32)")) -> (number=w274:u32)  [unwired: 1 in, 1 out]
                n69 = call "S7_Write.vi"("TCP"=w265, "寄存器类型"=w271, "DB #"=u16 20, "写入地址"=u32 2, "数据类型"=w270, "写入数据"=w274) -> ("TCP"=w267:refnum<k5>, "error out"=w268:errorcluster)  [unwired: 7 in, 1 out]
              }
              frame 3, Default {
                w289 = u8 132 items=["I/O (P)"=128, "Input (I)"=129, "Output (Q)"=130, "Bit Memory (M)"=131, "Data (DB)"=132, "Instance Data (DI)"=133, "Local Data (L)"=134, "Predecessor Local Data (VL)"=135] ("寄存器类型")
                w288 = u16 1 items=["byte", "word", "Dword"] ("数据类型")
                w296 = u8 132 items=["I/O (P)"=128, "Input (I)"=129, "Output (Q)"=130, "Bit Memory (M)"=131, "Data (DB)"=132, "Instance Data (DI)"=133, "Local Data (L)"=134, "Predecessor Local Data (VL)"=135] ("寄存器类型")
                w297 = u16 1 items=["byte", "word", "Dword"] ("数据类型")
                w303 = u8 132 items=["I/O (P)"=128, "Input (I)"=129, "Output (Q)"=130, "Bit Memory (M)"=131, "Data (DB)"=132, "Instance Data (DI)"=133, "Local Data (L)"=134, "Predecessor Local Data (VL)"=135] ("寄存器类型")
                w302 = u16 1 items=["byte", "word", "Dword"] ("数据类型")
                n70 = Index Array(array=w299) -> (element #1=w275:string, element #2=w282:string, element #3=w281:string)  [unwired: 3 in]
                n71 = Equal?(x=w281, y="OK") -> (x = y?=w279:bool)
                n72 = Decimal String To Number(string=w282, default (0L)=u32 0 ("默认(0 I32)")) -> (number=w283:u32)  [unwired: 1 in, 1 out]
                n73 = case shown="假" w279 {
                  tunnel: [u32 2 ("写入数据") u32 1 ("写入数据")] -> w278
                  frame False {
                  }
                  frame True {
                  }
                }
                n74 = call "S7_Write.vi"("TCP"=w286, "寄存器类型"=w303, "DB #"=u16 20, "写入地址"=u32 4, "数据类型"=w302, "写入数据"=w283) -> ("TCP"=w293:refnum<k5>, "error out"=w294:errorcluster)  [unwired: 7 in, 1 out]
                n75 = call "S7_Write.vi"("TCP"=w293, "寄存器类型"=w296, "DB #"=u16 20, "写入地址"=u32 6, "数据类型"=w297, "写入数据"=w278, "error in"=w294) -> ("TCP"=w285:refnum<k5>, "error out"=w284:errorcluster)  [unwired: 6 in, 1 out]
                n76 = Decimal String To Number(string=w275, default (0L)=u32 0 ("默认(0 I32)")) -> (number=w292:u32)  [unwired: 1 in, 1 out]
                n77 = call "S7_Write.vi"("TCP"=w285, "寄存器类型"=w289, "DB #"=u16 20, "写入地址"=u32 2, "数据类型"=w288, "写入数据"=w292, "error in"=w284) -> ("TCP"=w277:refnum<k5>, "error out"=w276:errorcluster)  [unwired: 6 in, 1 out]
              }
            }
            "扫码请求回复80" <- w255
            n78 = Bundle By Name(cluster=w257, "扫码超时"=w255) -> (w256:T5)
          }
          frame "-------------" {
          }
          frame "读扫码请求2" {
            w340 = u16 0 items=["byte", "word", "Dword"] ("数据类型")
            w342 = u8 132 items=["I/O (P)"=128, "Input (I)"=129, "Output (Q)"=130, "Bit Memory (M)"=131, "Data (DB)"=132, "Instance Data (DI)"=133, "Local Data (L)"=134, "Predecessor Local Data (VL)"=135] ("寄存器类型")
            n79 = call "S7_Read.vi"("TCP"=w332, "DB #"=u16 20, "读取长度"=u16 1, "寄存器类型"=w342, "起始地址"=u32 52, "数据类型"=w340) -> ("TCP"=w331:refnum<k5>, "数据"=w337:u32[], "error out"=w315:errorcluster)  [unwired: 6 in, 1 out]
            n80 = Index Array(array=w337, index=0 ("索引")) -> (element=w335:u32)
            n81 = Number To Boolean Array(number=w335) -> (Boolean array=w334:bool[])
            n82 = Index Array(array=w334, index=0 ("索引")) -> (element=w313:bool)
            "ST802扫码请求" <- w313
            n83 = Unbundle By Name(w316) -> ("扫码超时 2"=w318:string)
            n84 = Not Equal?(x=w318, y="999") -> (x != y?=w320:bool)
            n85 = call <vilib>:"Boolean Crossing PtByPt.vi"("direction"=enum16{"either", "false-true", "true-false"}."true-false", "input"=w313) -> ("crossing"=w312:bool)  [unwired: 1 in]
            n86 = call <vilib>:"Boolean Crossing PtByPt.vi"("direction"=enum16{"either", "false-true", "true-false"}."false-true", "input"=w313) -> ("crossing"=w328:bool)  [unwired: 1 in]
            n87 = Not(x=w320) -> (.not. x?=w321:bool)
            n88 = call "已用时间30"("Reset"=w321) -> ("Time has Elapsed"=w322:bool)  [unwired: 11 in, 7 out]
            n89 = Insert Into Array(array=bool[] [] ("数组"), index=0 ("索引"), new element #1=w328, new element #2=w312) -> (w325:bool[])
            n90 = Boolean Array To Number(Boolean array=w325) -> (number=w324:u32)
            n91 = case shown="2" w324 {
              tunnel: [cluster{"Data":string[], "State":T1} {"Data"=[], "State"=enum."读数据保存请求2"} ("元素") w347 w351] -> w323
              tunnel: w317 -> [_ w348 w352]
              frame 0, Default {
              }
              frame 1 {
                w347 = cluster{"Data":string[], "State":T1} {"Data"=[], "State"=enum."读二维码2"} ("元素")
                n92 = Enqueue Element(queue=w348, element=w347, timeout in ms (-1)=10 ("超时毫秒(-1)")) -> ()  [unwired: 1 in, 3 out]
              }
              frame 2 {
                w351 = cluster{"Data":string[], "State":T1} {"Data"=["999"], "State"=enum."扫码回复2"} ("元素")
                n93 = Enqueue Element(queue=w352, element=w351, timeout in ms (-1)=10 ("超时毫秒(-1)")) -> ()  [unwired: 1 in, 3 out]
              }
            }
            n94 = case shown="真" w322 {
              tunnel: w317 -> [_ w344]
              frame False {
              }
              frame True {
                n95 = Enqueue Element(queue=w344, element=cluster{"Data":string[], "State":T1} {"Data"=["999"], "State"=enum."扫码回复2"} ("元素"), timeout in ms (-1)=10 ("超时毫秒(-1)")) -> ()  [unwired: 1 in, 3 out]
              }
            }
          }
          frame "读二维码2" {
            w371 = u16 0 items=["byte", "word", "Dword"] ("数据类型")
            w367 = u8 132 items=["I/O (P)"=128, "Input (I)"=129, "Output (Q)"=130, "Bit Memory (M)"=131, "Data (DB)"=132, "Instance Data (DI)"=133, "Local Data (L)"=134, "Predecessor Local Data (VL)"=135] ("寄存器类型")
            n96 = call "S7_Read.vi"("TCP"=w362, "DB #"=u16 20, "读取长度"=u16 17, "寄存器类型"=w367, "起始地址"=u32 10, "数据类型"=w371) -> ("TCP"=w366:refnum<k5>, "数据"=w372:u32[], "读取成功"=w360:bool, "error out"=w374:errorcluster)  [unwired: 6 in]
            n97 = disable-structure shown="禁用" {
              frame Disabled {
                n98 = String Subset(offset (0)=0 ("偏移量(0)"), length (rest)=13 ("长度（剩余）")) -> ()  [unwired: 1 in, 1 out]
              }
              frame Enabled {
              }
            }
            n99 = Not(x=w360) -> (.not. x?=w361:bool)
            n100 = To Unsigned Word Integer(number=w372) -> (unsigned 16bit integer=w373:u16[])
            n101 = local write "ST80通讯状态"(w361) -> ()
            n102 = call "还原为字符串.vi"("error in (no error)"=w374, "输入数组"=w373) -> ("error out"=w358:errorcluster, "字符串"=w354:string)  [unwired: 8 in]
            n103 = String Subset(string=w354, offset (0)=0 ("偏移量(0)"), length (rest)=13 ("长度（剩余）")) -> (substring=w353:string)
            n104 = flat-sequence {
              tunnel: w353 -> [w378]
              tunnel: w358 -> [w377]
              tunnel: [w377] -> w357
              tunnel: [w380] -> w359
              tunnel: w357 -> [w379]
              frame #0 {
                "802二维码" <- w378
              }
              frame #1 {
                n105 = property on="ST802扫码请求(事件)" class="Bool (严格)"(error in=w379, "Val(Sgnl)"=TRUE ("值(信号)")) -> (error out=w380:errorcluster)  [unwired: 1 in, 1 out]
              }
            }
          }
          frame "扫码回复2" {
            n106 = Array Size(array=w386) -> (size(s)=w387:i32)
            n107 = case shown="3, 默认" w387 {
              tunnel: w386 -> [w394 w427]
              tunnel: w389 -> [w393 w414]
              tunnel: [w395 w405] -> w388
              tunnel: [w396 w404] -> w383
              tunnel: [w392 w403] -> w382
              frame 1 {
                w399 = u8 132 items=["I/O (P)"=128, "Input (I)"=129, "Output (Q)"=130, "Bit Memory (M)"=131, "Data (DB)"=132, "Instance Data (DI)"=133, "Local Data (L)"=134, "Predecessor Local Data (VL)"=135] ("寄存器类型")
                w398 = u16 1 items=["byte", "word", "Dword"] ("数据类型")
                n108 = Index Array(array=w394) -> (element=w392:string)  [unwired: 1 in]
                n109 = Decimal String To Number(string=w392, default (0L)=u32 0 ("默认(0 I32)")) -> (number=w402:u32)  [unwired: 1 in, 1 out]
                n110 = call "S7_Write.vi"("TCP"=w393, "寄存器类型"=w399, "DB #"=u16 20, "写入地址"=u32 54, "数据类型"=w398, "写入数据"=w402) -> ("TCP"=w395:refnum<k5>, "error out"=w396:errorcluster)  [unwired: 7 in, 1 out]
              }
              frame 3, Default {
                w417 = u8 132 items=["I/O (P)"=128, "Input (I)"=129, "Output (Q)"=130, "Bit Memory (M)"=131, "Data (DB)"=132, "Instance Data (DI)"=133, "Local Data (L)"=134, "Predecessor Local Data (VL)"=135] ("寄存器类型")
                w416 = u16 1 items=["byte", "word", "Dword"] ("数据类型")
                w424 = u8 132 items=["I/O (P)"=128, "Input (I)"=129, "Output (Q)"=130, "Bit Memory (M)"=131, "Data (DB)"=132, "Instance Data (DI)"=133, "Local Data (L)"=134, "Predecessor Local Data (VL)"=135] ("寄存器类型")
                w425 = u16 1 items=["byte", "word", "Dword"] ("数据类型")
                w431 = u8 132 items=["I/O (P)"=128, "Input (I)"=129, "Output (Q)"=130, "Bit Memory (M)"=131, "Data (DB)"=132, "Instance Data (DI)"=133, "Local Data (L)"=134, "Predecessor Local Data (VL)"=135] ("寄存器类型")
                w430 = u16 1 items=["byte", "word", "Dword"] ("数据类型")
                n111 = Index Array(array=w427) -> (element #1=w403:string, element #2=w410:string, element #3=w409:string)  [unwired: 3 in]
                n112 = Equal?(x=w409, y="OK") -> (x = y?=w407:bool)
                n113 = Decimal String To Number(string=w410, default (0L)=u32 0 ("默认(0 I32)")) -> (number=w411:u32)  [unwired: 1 in, 1 out]
                n114 = case shown="假" w407 {
                  tunnel: [u32 2 ("写入数据") u32 1 ("写入数据")] -> w406
                  frame False {
                  }
                  frame True {
                  }
                }
                n115 = call "S7_Write.vi"("TCP"=w414, "寄存器类型"=w431, "DB #"=u16 20, "写入地址"=u32 4, "数据类型"=w430, "写入数据"=w411) -> ("TCP"=w421:refnum<k5>, "error out"=w422:errorcluster)  [unwired: 7 in, 1 out]
                n116 = call "S7_Write.vi"("TCP"=w421, "寄存器类型"=w424, "DB #"=u16 20, "写入地址"=u32 6, "数据类型"=w425, "写入数据"=w406, "error in"=w422) -> ("TCP"=w413:refnum<k5>, "error out"=w412:errorcluster)  [unwired: 6 in, 1 out]
                n117 = Decimal String To Number(string=w403, default (0L)=u32 0 ("默认(0 I32)")) -> (number=w420:u32)  [unwired: 1 in, 1 out]
                n118 = call "S7_Write.vi"("TCP"=w413, "寄存器类型"=w417, "DB #"=u16 20, "写入地址"=u32 54, "数据类型"=w416, "写入数据"=w420, "error in"=w412) -> ("TCP"=w405:refnum<k5>, "error out"=w404:errorcluster)  [unwired: 6 in, 1 out]
              }
            }
            n119 = Bundle By Name(cluster=w385, "扫码超时 2"=w382) -> (w384:T5)
            n120 = local write "80保存回复"(w382) -> ()
          }
          frame "-- --------------" {
          }
          frame "读数据保存请求2" {
            w468 = u16 0 items=["byte", "word", "Dword"] ("数据类型")
            w470 = u8 132 items=["I/O (P)"=128, "Input (I)"=129, "Output (Q)"=130, "Bit Memory (M)"=131, "Data (DB)"=132, "Instance Data (DI)"=133, "Local Data (L)"=134, "Predecessor Local Data (VL)"=135] ("寄存器类型")
            n121 = call "S7_Read.vi"("TCP"=w460, "DB #"=u16 20, "读取长度"=u16 1, "寄存器类型"=w470, "起始地址"=u32 56, "数据类型"=w468) -> ("TCP"=w459:refnum<k5>, "数据"=w465:u32[], "error out"=w443:errorcluster)  [unwired: 6 in, 1 out]
            n122 = Index Array(array=w465, index=0 ("索引")) -> (element=w463:u32)
            n123 = Number To Boolean Array(number=w463) -> (Boolean array=w462:bool[])
            n124 = Index Array(array=w462, index=0 ("索引")) -> (element=w441:bool)
            "ST802保存数据" <- w441
            n125 = Unbundle By Name(w444) -> ("数据保存超时"=w446:string)
            n126 = Not Equal?(x=w446, y="999") -> (x != y?=w448:bool)
            n127 = call <vilib>:"Boolean Crossing PtByPt.vi"("direction"=enum16{"either", "false-true", "true-false"}."false-true", "input"=w441) -> ("crossing"=w456:bool)  [unwired: 1 in]
            n128 = call <vilib>:"Boolean Crossing PtByPt.vi"("direction"=enum16{"either", "false-true", "true-false"}."true-false", "input"=w441) -> ("crossing"=w440:bool)  [unwired: 1 in]
            n129 = Not(x=w448) -> (.not. x?=w449:bool)
            n130 = call "已用时间31"("Reset"=w449) -> ("Time has Elapsed"=w450:bool)  [unwired: 11 in, 7 out]
            n131 = Insert Into Array(array=bool[] [] ("数组"), index=0 ("索引"), new element #1=w456, new element #2=w440) -> (w453:bool[])
            n132 = Boolean Array To Number(Boolean array=w453) -> (number=w452:u32)
            n133 = case shown="2" w452 {
              tunnel: [cluster{"Data":string[], "State":T1} {"Data"=[], "State"=enum."看门狗"} ("元素") w475 w479] -> w451
              tunnel: w445 -> [_ w476 w480]
              frame 0, Default {
              }
              frame 1 {
                w475 = cluster{"Data":string[], "State":T1} {"Data"=[], "State"=enum."读数据2"} ("元素")
                n134 = Enqueue Element(queue=w476, element=w475, timeout in ms (-1)=10 ("超时毫秒(-1)")) -> ()  [unwired: 1 in, 3 out]
              }
              frame 2 {
                w479 = cluster{"Data":string[], "State":T1} {"Data"=["999"], "State"=enum."数据保存回复2"} ("元素")
                n135 = Enqueue Element(queue=w480, element=w479, timeout in ms (-1)=10 ("超时毫秒(-1)")) -> ()  [unwired: 1 in, 3 out]
              }
            }
            n136 = case shown="真" w450 {
              tunnel: w445 -> [_ w472]
              frame False {
              }
              frame True {
                n137 = Enqueue Element(queue=w472, element=cluster{"Data":string[], "State":T1} {"Data"=["999"], "State"=enum."数据保存回复2"} ("元素"), timeout in ms (-1)=10 ("超时毫秒(-1)")) -> ()  [unwired: 1 in, 3 out]
              }
            }
          }
          frame "读数据2" {
            w492 = u16 1 items=["byte", "word", "Dword"] ("数据类型")
            w494 = u8 132 items=["I/O (P)"=128, "Input (I)"=129, "Output (Q)"=130, "Bit Memory (M)"=131, "Data (DB)"=132, "Instance Data (DI)"=133, "Local Data (L)"=134, "Predecessor Local Data (VL)"=135] ("寄存器类型")
            w515 = u16 0 items=["byte", "word", "Dword"] ("数据类型")
            w500 = u16 20 ("DB #")
            w512 = u8 132 items=["I/O (P)"=128, "Input (I)"=129, "Output (Q)"=130, "Bit Memory (M)"=131, "Data (DB)"=132, "Instance Data (DI)"=133, "Local Data (L)"=134, "Predecessor Local Data (VL)"=135] ("寄存器类型")
            n138 = call "S7_Read.vi"("TCP"=w509, "DB #"=w500, "读取长度"=u16 19, "寄存器类型"=w512, "起始地址"=u32 28, "数据类型"=w515) -> ("TCP"=w498:refnum<k5>, "数据"=w516:u32[], "读取成功"=w507:bool, "error out"=w497:errorcluster)  [unwired: 6 in]
            n139 = Not(x=w507) -> (.not. x?=w508:bool)
            n140 = local write "ST80通讯状态"(w508) -> ()
            n141 = To Unsigned Word Integer(number=w516) -> (unsigned 16bit integer=w517:u16[])
            n142 = call "还原为字符串.vi"("输入数组"=w517) -> ("字符串"=w504:string)  [unwired: 9 in, 1 out]
            n143 = call "S7_Read.vi"("TCP"=w498, "DB #"=w500, "读取长度"=u16 1, "寄存器类型"=w494, "起始地址"=u32 60, "数据类型"=w492, "error in"=w497) -> ("TCP"=w495:refnum<k5>, "数据"=w491:u32[], "error out"=w496:errorcluster)  [unwired: 5 in, 1 out]
            n144 = String Subset(string=w504, offset (0)=18 ("偏移量(0)"), length (rest)=1 ("长度（剩余）")) -> (substring=w483:string)
            n145 = String Subset(string=w504, offset (0)=0 ("偏移量(0)"), length (rest)=17 ("长度（剩余）")) -> (substring=w484:string)
            n146 = Index Array(array=w491) -> (element=w490:u32)  [unwired: 1 in]
            n147 = Equal?(x=w490, y=u32 1) -> (x = y?=w488:bool)
            n148 = Select(t="OK", s=w488, f="NG") -> (s? t:f=w485:string)
            n149 = flat-sequence {
              tunnel: w496 -> [w528]
              tunnel: [w528] -> w501
              tunnel: w485 -> [w524]
              tunnel: w484 -> [w520]
              tunnel: w483 -> [w519]
              tunnel: [w530] -> w482
              tunnel: w501 -> [w529]
              frame #0 {
                n150 = Format Date/Time String(time format string (%c)="%Y-%m-%d" ("时间格式字符串(%c)")) -> (date/time string=w522:string)  [unwired: 2 in]
                n151 = Get Date/Time String() -> (time string=w521:string)  [unwired: 3 in, 1 out]
                n152 = Insert Into Array(array=string[] [], index=0 ("索引"), new element #1="80", new element #2=w524, new element #3=w522, new element #4=w521, new element #5=w520, new element #6=w519) -> (→"802数据":string[])
              }
              frame #1 {
                n153 = property on="ST802保存数据(事件)" class="Bool (严格)"(error in=w529, "Val(Sgnl)"=TRUE ("值(信号)")) -> (error out=w530:errorcluster)  [unwired: 1 in, 1 out]
              }
            }
          }
          frame "数据保存回复2" {
            w541 = u8 132 items=["I/O (P)"=128, "Input (I)"=129, "Output (Q)"=130, "Bit Memory (M)"=131, "Data (DB)"=132, "Instance Data (DI)"=133, "Local Data (L)"=134, "Predecessor Local Data (VL)"=135] ("寄存器类型")
            w542 = u16 1 items=["byte", "word", "Dword"] ("数据类型")
            n154 = Index Array(array=w536, index=0 ("索引")) -> (element=w532:string)
            "80保存回复" <- w532
